vi "Current VI's Path in Different APP Kind__Uti.vi"() -> (4 "Config":path, 5 "Files":path, 7 "Measure":path, 8 "Cursor":path)   [LabVIEW 2012]
doc: "得到当前VI的路径和relative path(.)端口的组合路径.\n这个VI解决了LabVIEW自带函数调试环境下和编译环境下输出不一样的Bug\n\nControls\nrelative path (.): 相对路径\n\nIndicators\ncurrent VI's path + relative path:得到当前VI的路径和relative path(.)端口的组合路径"
panel:
  # "得到当前VI的路径和relative path(.)端口的组合路径.\n这个VI解决了LabVIEW自带函数调试环境下和编译环境下输出不一样的Bug\n\nControls\nrelative path (.): 相对路径\n\nIndicators\ncurrent VI's path + relative path:得到当前VI的路径和relative path(.)端口的组合路径"
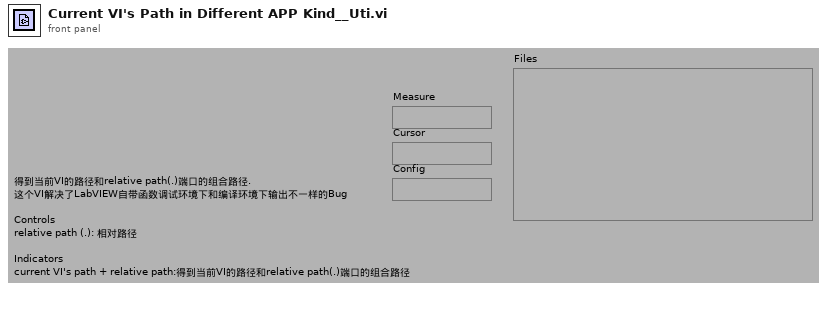
[diagram p1: front panel]
types:
  T1 = enum32{"invalid app kind", "Development System", "Run Time System", "Student Edition", "Embedded LabVIEW", "Evaluation", "Custom"}
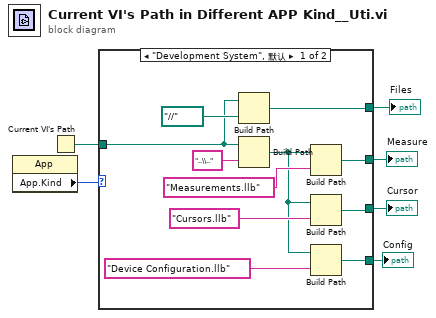
[diagram p0: block diagram]
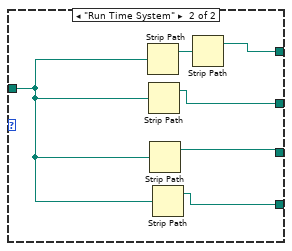
[diagram p2: hidden frame]
diagram:
  n1 = property class="App"() -> ("App.Kind"=w1:T1)  [unwired: 2 in, 2 out]
  n2 = Current VI's Path() -> (path=w6:path)
  n3 = case shown="\"Development System\", 默认" w1 {
    tunnel: [w15 w22] -> w4
    tunnel: [w13 w21] -> w3
    tunnel: w6 -> [w11 w20]
    tunnel: [w10 w18] -> w5
    tunnel: [w7 w19] -> w2
    frame "Development System", Default {
      n4 = Build Path(base path=w11, name or relative path=path "../../.." ("relative path (.)")) -> (appended path=w10:path)
      n5 = Build Path(base path=w11, name or relative path="..\\..") -> (appended path=w9:path)
      n6 = Build Path(base path=w9, name or relative path="Measurements.llb") -> (appended path=w15:path)
      n7 = Build Path(base path=w9, name or relative path="Cursors.llb") -> (appended path=w13:path)
      n8 = Build Path(base path=w9, name or relative path="Device Configuration.llb") -> (appended path=w7:path)
    }
    frame "Run Time System" {
      n9 = Strip Path(path=w20) -> (stripped path=w23:path)  [unwired: 1 out]
      n10 = Strip Path(path=w20) -> (stripped path=w22:path)  [unwired: 1 out]
      n11 = Strip Path(path=w20) -> (stripped path=w21:path)  [unwired: 1 out]
      n12 = Strip Path(path=w20) -> (stripped path=w19:path)  [unwired: 1 out]
      n13 = Strip Path(path=w23) -> (stripped path=w18:path)  [unwired: 1 out]
    }
  }
  "Files" <- w5
  "Measure" <- w4
  "Cursor" <- w3
  "Config" <- w2
